vi "Numeric converter helper.vi"() -> ()   [LabVIEW 2022 SP3]
panel:
  in  "8-bit binary in":bool[](array[boolean])=[TRUE, TRUE, TRUE, TRUE, TRUE, TRUE, TRUE, TRUE]
  out "Hex out":u8=255 format="%02x"
  out "Dec out":u8=255 format="%03.0f"
  out "Hex checksum":u8=195 format="%02x"
  out "binary":string="11000000"
  out "8-bit binary":bool[](array[boolean])=[TRUE, TRUE, FALSE, FALSE, FALSE, FALSE, FALSE, FALSE]
  out "8-bit binary":bool[](array[boolean])=[TRUE, TRUE, TRUE, FALSE, TRUE, FALSE, TRUE, TRUE]
  out "binary":string="11101011"
  out "Hex out":u8=235 format="%02x"
  in  "Dec in":u8=235 step=1 format="%03d"
  out "Dec out":u8=192 format="%03.0f"
  in  "Hex in":u8=192 step=1 format="%02x"
  in  "String":string="!010806C0"
  # "to"
  # "MSB"
  # "LSB"
  # "to"
  # "MSB"
  # "LSB"
  # "to"
  # "MSB"
  # "LSB"
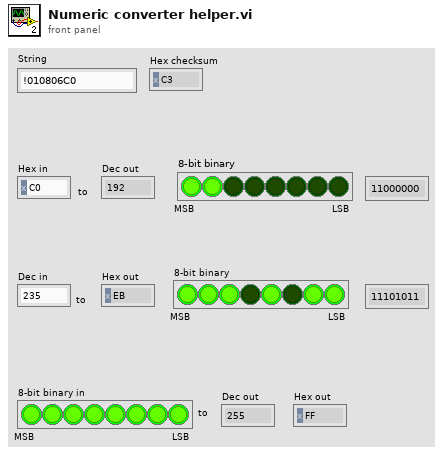
[diagram p1: front panel]
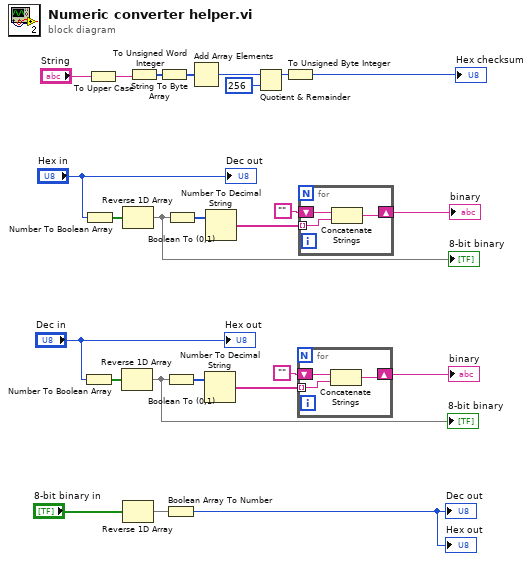
[diagram p0: block diagram]
diagram:
  n1 = Number To Boolean Array(number="Dec in") -> (Boolean array=w21:bool[])
  n2 = Number To Boolean Array(number="Hex in") -> (Boolean array=w16:bool[])
  n3 = To Upper Case(1:"String") -> (0:w6:string)
  n4 = Reverse 1D Array(array=w21) -> (reversed array=w20:bool[])
  "8-bit binary" <- w20
  n5 = Reverse 1D Array(array=w16) -> (reversed array=w17:bool[])
  "8-bit binary" <- w17
  n6 = Reverse 1D Array(array="8-bit binary in") -> (reversed array=w1:bool[])
  n7 = String To Byte Array(string=w6) -> (unsigned byte array=w9:u8[])
  n8 = To Unsigned Word Integer(number=w9) -> (unsigned 16bit integer=w8:u16[])
  n9 = Boolean To (0,1)(Boolean=w20) -> (0, 1=w24:i16[])
  n10 = Boolean Array To Number(Boolean array=w1) -> (number=→"Dec out" →"Hex out":u32)
  n11 = Boolean To (0,1)(Boolean=w17) -> (0, 1=w13:i16[])
  n12 = Add Array Elements(numeric array=w8) -> (sum=w7:u16)
  n13 = Number To Decimal String(number=w24) -> (decimal integer string=w19:string[])  [unwired: 1 in]
  n14 = Number To Decimal String(number=w13) -> (decimal integer string=w18:string[])  [unwired: 1 in]
  n15 = Quotient & Remainder(x=w7, y=u16 256) -> (x-y*floor(x/y)=w10:u16)  [unwired: 1 out]
  n16 = To Unsigned Byte Integer(number=w10) -> (unsigned 8bit integer=→"Hex checksum":u8)
  n17 = for {
    tunnel: w19 -> [w26] mode=indexing
    shift-right: [w27] -> w22
    shift-left: "" -> [w28]
    n18 = Concatenate Strings(w28, w26) -> (w27:string)
  }
  "binary" <- w22
  n19 = for {
    tunnel: w18 -> [w29] mode=indexing
    shift-right: [w30] -> w15
    shift-left: "" -> [w31]
    n20 = Concatenate Strings(w31, w29) -> (w30:string)
  }
  "binary" <- w15
  "Dec out" <- "Hex in"
  "Hex out" <- "Dec in"
